vi "BSA output Freq Shift.vi"(3 "BSAIP__ChNum":string[](array[string])) -> (0 "BSA Error":errorcluster)   [LabVIEW 2020]
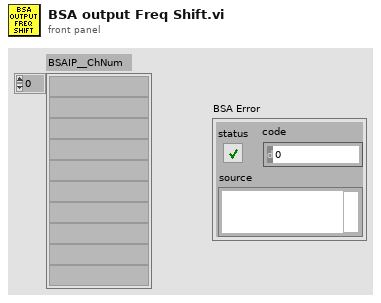
[diagram p1: front panel]
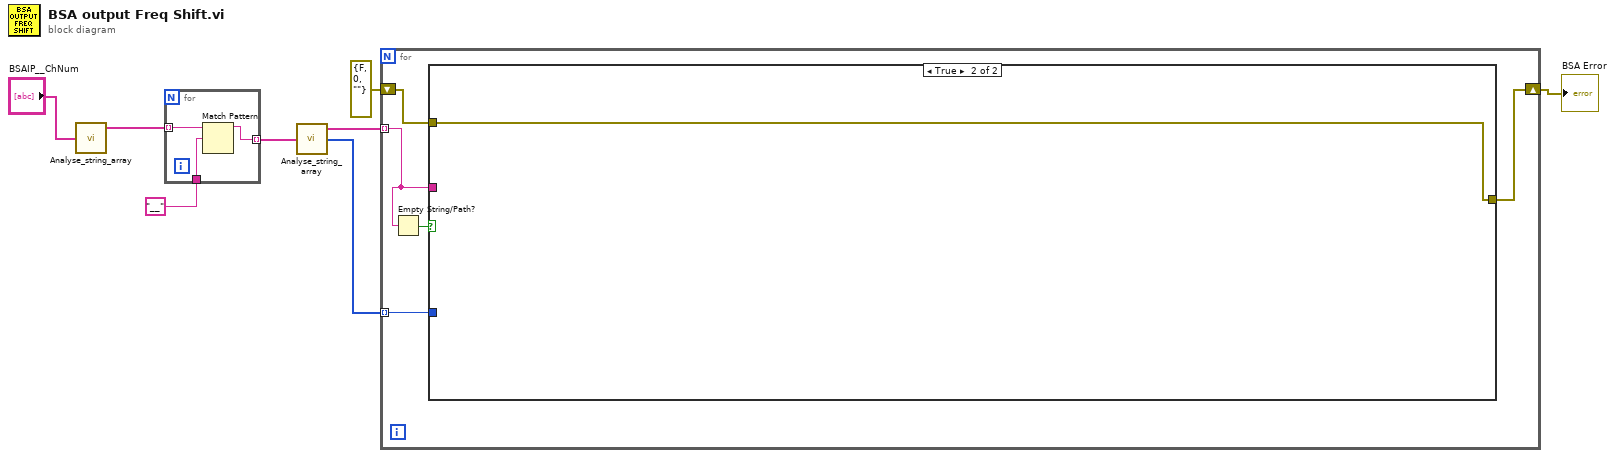
[diagram p0: block diagram]
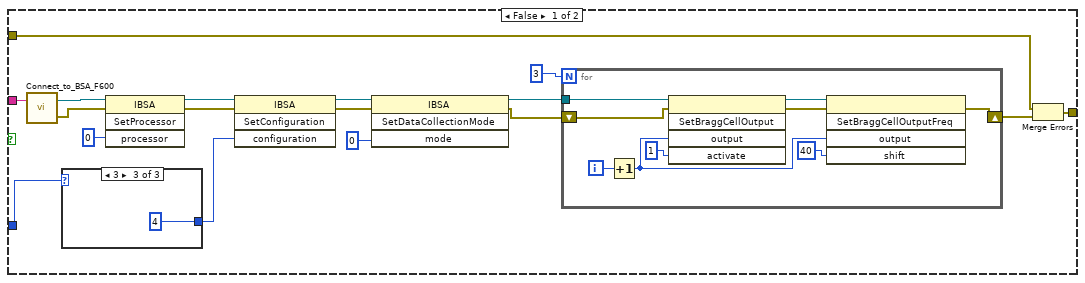
[diagram p2: hidden frame]
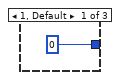
[diagram p3: hidden frame]
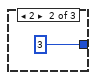
[diagram p4: hidden frame]
diagram:
  n1 = call "Analyse_string_array.vi"("String array"="BSAIP__ChNum") -> ("Unique strings"=w7:string[])  [unwired: 1 in, 1 out]
  n2 = for {
    tunnel: "__" ("string") -> [w11]
    tunnel: w7 -> [w10] mode=indexing
    tunnel: [w9] -> w8 mode=indexing
    n3 = Match Pattern(string=w10, regular expression=w11) -> (before substring=w9:string)  [unwired: 1 in, 3 out]
  }
  n4 = call "Analyse_string_array.vi"("String array"=w8) -> ("Unique strings"=w5:string[], "Frequency"=w4:i32[])  [unwired: 1 in]
  n5 = for {
    tunnel: w5 -> [w13] mode=indexing
    tunnel: w4 -> [w16] mode=indexing
    shift-right: [w14] -> w2
    shift-left: errorcluster {"status"=FALSE, "code"=0, "source"=""} ("error IO") -> [w15]
    n6 = Empty String/Path?(string/path=w13) -> (empty?=w12:bool)
    n7 = case shown="True" w12 {
      tunnel: w13 -> [w22 _]
      tunnel: w16 -> [w21 _]
      tunnel: w15 -> [w18 w46]
      tunnel: [w17 w46] -> w14
      frame False {
        n8 = call "Connect_to_BSA_F600.vi"("BSA IP Number"=w22) -> ("error out"=w28:errorcluster, "F600"=w27:refnum<k7>)  [unwired: 1 in]
        n9 = case shown="3" w21 {
          tunnel: [0 ("configuration") 3 ("configuration") 4 ("configuration")] -> w20
          frame 1, Default {
          }
          frame 2 {
          }
          frame 3 {
          }
        }
        n10 = invoke class="IBSA" method="SetProcessor"(reference=w27, error in=w28, "processor"=0) -> (reference out=w25:refnum<k7>, error out=w24:errorcluster)  [unwired: 1 in, 2 out]
        n11 = invoke class="IBSA" method="SetConfiguration"(reference=w25, error in=w24, "configuration"=w20) -> (reference out=w30:refnum<k7>, error out=w32:errorcluster)  [unwired: 1 in, 2 out]
        n12 = invoke class="IBSA" method="SetDataCollectionMode"(reference=w30, error in=w32, "mode"=0) -> (reference out=w31:refnum<k7>, error out=w33:errorcluster)  [unwired: 1 in, 2 out]
        n13 = for {
          N: 3 -> [_]
          tunnel: w31 -> [w41]
          shift-right: [w37] -> w19
          shift-left: w33 -> [w38]
          i -> [w40]
          n14 = Increment(x=w40) -> (x+1=w45:i32)
          n15 = invoke method="SetBraggCellOutput"(reference=w41, error in=w38, "output"=w45, "activate"=1) -> (reference out=w43:refnum<k7>, error out=w44:errorcluster)  [unwired: 1 in, 3 out]
          n16 = invoke method="SetBraggCellOutputFreq"(reference=w43, error in=w44, "output"=w45, "shift"=40) -> (error out=w37:errorcluster)  [unwired: 1 in, 4 out]
        }
        n17 = Merge Errors(w18, w19) -> (w17:errorcluster)
      }
      frame True {
      }
    }
  }
  "BSA Error" <- w2
